vi "Chi-Squared (Non-Central) CDF.vi"(9 "d":dbl, 10 "k":i32=1, 11 "x":dbl=1.0) -> (0 "error":i32, 3 "cdf(x)":dbl=0.682689492137086)   [LabVIEW 2017, in "NI_Gmath.lvlib"]
doc: "Computes the continuous cumulative distribution function (CDF), or the probability that the random variate X, where X describes the selected distribution type, has a value less than or equal to <B>x</B>. You must manually select the polymorphic instance to use."
uses:
  <vilib>/gmath/NI_Gmath.lvlib
  <vilib>/gmath/statdist.llb/st_error_code.ctl
  <vilib>/gmath/SpecialFunctions.llb/Incomplete Gamma Function.vi
panel:
  # "Chi-Squared (Non-Central) CDF"
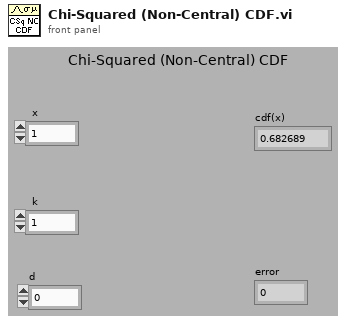
[diagram p1: front panel]
types:
  T1 = typedef "NI_Gmath.lvlib/st_error_code.ctl" = i32
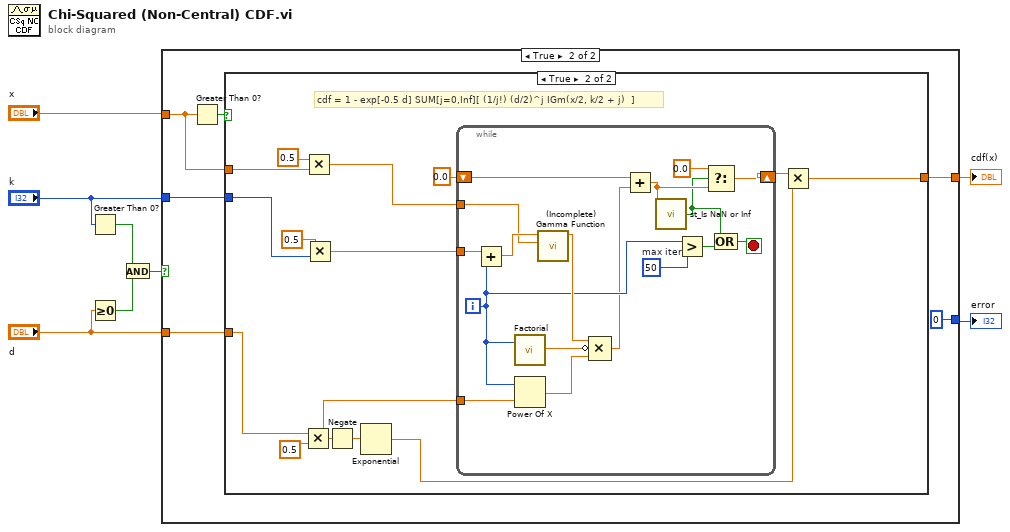
[diagram p0: block diagram]
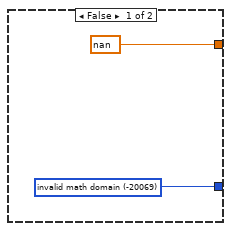
[diagram p2: hidden frame]
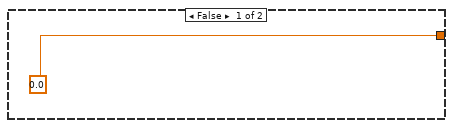
[diagram p3: hidden frame]
diagram:
  n1 = Greater Than 0?(x="k") -> (x > 0?=w3:bool)
  n2 = Greater Or Equal To 0?(x="d") -> (x >= 0?=w4:bool)
  n3 = And(x=w3, y=w4) -> (x .and. y?=w8:bool)
  n4 = case shown="True" w8 {
    tunnel: [w9 0 ("invalid math domain")] -> w7
    tunnel: [nan w15] -> w2
    tunnel: "x" -> [_ w13]
    tunnel: "k" -> [_ w14]
    tunnel: "d" -> [_ w11]
    frame False {
      w9 = T1 -20069 items=["invalid math domain"=-20069, "Fourier interpolation size m >= n"=-20070, "empty array"=-20003] ("stat interp error code")
    }
    frame True {
      n5 = Greater Than 0?(x=w13) -> (x > 0?=w12:bool)
      n6 = case shown="True" w12 {
        tunnel: [0.0 w18] -> w15
        tunnel: w13 -> [_ w25]
        tunnel: w14 -> [_ w31]
        tunnel: w11 -> [_ w26]
        frame False {
        }
        frame True {
          # "cdf = 1 - exp[-0.5 d] SUM[j=0,Inf][ (1/j!) (d/2)^j IGm(x/2, k/2 + j)  ]"
          n7 = Multiply(x=w26, y=0.5 ("x")) -> (x*y=w21:dbl)
          n8 = Multiply(x=0.5, y=w25) -> (x*y=w23:dbl)
          n9 = Multiply(x=0.5, y=w31) -> (x*y=w27:dbl)
          n10 = Negate(x=w21) -> (-x=w22:dbl)
          n11 = Exponential(1:w22) -> (0:w19:dbl)
          n12 = while {
            shift-right: [w44] -> w20
            shift-left: 0.0 ("x") -> [w47]
            tunnel: w27 -> [w48]
            tunnel: w23 -> [w32]
            tunnel: w21 -> [w33]
            i -> [w40]
            stop <- w41 stop-if-true
            w37 = 50  # max iter
            n13 = Add(x=w48, y=w40) -> (x+y=w34:dbl)
            n14 = call <vilib>:"Factorial.vi"("n"=w40) -> ("n!"=w43:dbl)  [unwired: 2 in]
            n15 = Power Of X(1:w33, 2:w40) -> (0:w35:dbl)
            n16 = call-poly <vilib>:"(Incomplete) Gamma Function.vi"("a"=w32, "x"=w34) -> ("g(x, a)"=w42:dbl)  [unwired: 9 in]
            n17 = Compound Arithmetic op=MULTIPLY(w42, invert w43, w35) -> (w36:dbl)
            n18 = Add(x=w47, y=w36) -> (x+y=w45:dbl)
            n19 = call <vilib>:"st_Is NaN or Inf.vi"("x"=w45) -> ("isNaN(x) || isInf(x)"=w38:bool)  [unwired: 4 in]
            n20 = Greater?(x=w40, y=w37) -> (0:w39:bool)
            n21 = Select(t=0.0, s=w38, f=w45) -> (s? t:f=w44:dbl)
            n22 = Compound Arithmetic op=OR(w38, w39) -> (w41:bool)
          }
          n23 = Multiply(x=w20, y=w19) -> (x*y=w18:dbl)
        }
      }
    }
  }
  "cdf(x)" <- w2
  "error" <- w7
